vi "oa_SCL Calc Shaft Axis Max Min Value.vi"(0 "clearance boundary settings":T1) -> (1 "x axis max":dbl, 2 "x axis min":dbl, 3 "y axis max":dbl, 4 "y axis min":dbl)   [LabVIEW 2017]
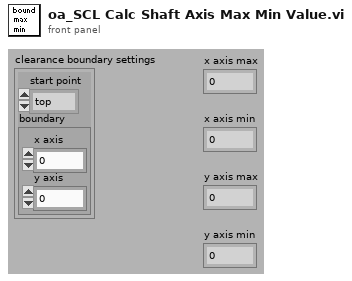
[diagram p1: front panel]
types:
  T1 = cluster{"start point":enum16{"top", "center", "bottom"}, "boundary":cluster{"x axis":dbl, "y axis":dbl}}
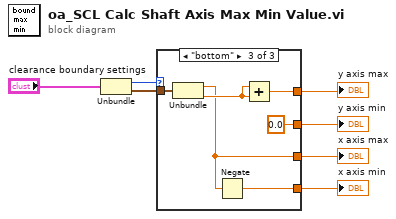
[diagram p0: block diagram]
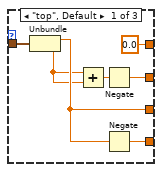
[diagram p2: hidden frame]
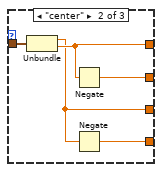
[diagram p3: hidden frame]
diagram:
  n1 = Unbundle("clearance boundary settings") -> ("start point"=w6:enum16{"top", "center", "bottom"}, "boundary"=w7:cluster{"x axis":dbl, "y axis":dbl})
  n2 = case shown="\"bottom\"" w6 {
    tunnel: w7 -> [w14 w19 w25]
    tunnel: [0.0 w16 w24] -> w4
    tunnel: [w11 w18 0.0] -> w2
    tunnel: [w9 w15 w20] -> w3
    tunnel: [w10 w17 w23] -> w1
    frame "top", Default {
      n3 = Unbundle(w14) -> ("x axis"=w9:dbl, "y axis"=w8:dbl)
      n4 = Add(x=w8, y=w8) -> (x+y=w13:dbl)
      n5 = Negate(x=w13) -> (-x=w11:dbl)
      n6 = Negate(x=w9) -> (-x=w10:dbl)
    }
    frame "center" {
      n7 = Unbundle(w19) -> ("x axis"=w15:dbl, "y axis"=w16:dbl)
      n8 = Negate(x=w16) -> (-x=w18:dbl)
      n9 = Negate(x=w15) -> (-x=w17:dbl)
    }
    frame "bottom" {
      n10 = Unbundle(w25) -> ("x axis"=w20:dbl, "y axis"=w21:dbl)
      n11 = Negate(x=w20) -> (-x=w23:dbl)
      n12 = Add(x=w21, y=w21) -> (x+y=w24:dbl)
    }
  }
  "y axis min" <- w2
  "y axis max" <- w4
  "x axis min" <- w1
  "x axis max" <- w3
